vi "SDCP Receiver and Transmitter - Tx Table.vi"(5 "Cell Position":T2, 7 "Table Control":refnum<vi>, 8 "error in (no error)":errorcluster, 9 "Command":T3(ring), 10 "FID":i32, 11 "SMF Parameters descriptors":T4[](array[typedef])) -> (0 "error out":errorcluster, 3 "Table elements out":T1[](array[typedef]))   [LabVIEW 2020]
uses:
  Typedefs/SDCP - SMF parameter descriptors.ctl
  <vilib>/Utility/miscctls.llb/LVRowAndColumnTypeDef.ctl
  Typedefs/SDCP SMF Receiver and Transmitter - Transmit Table Element.ctl
  Typedefs/SDCP - Standard Message Frame Parameters - FGV - commands.ctl
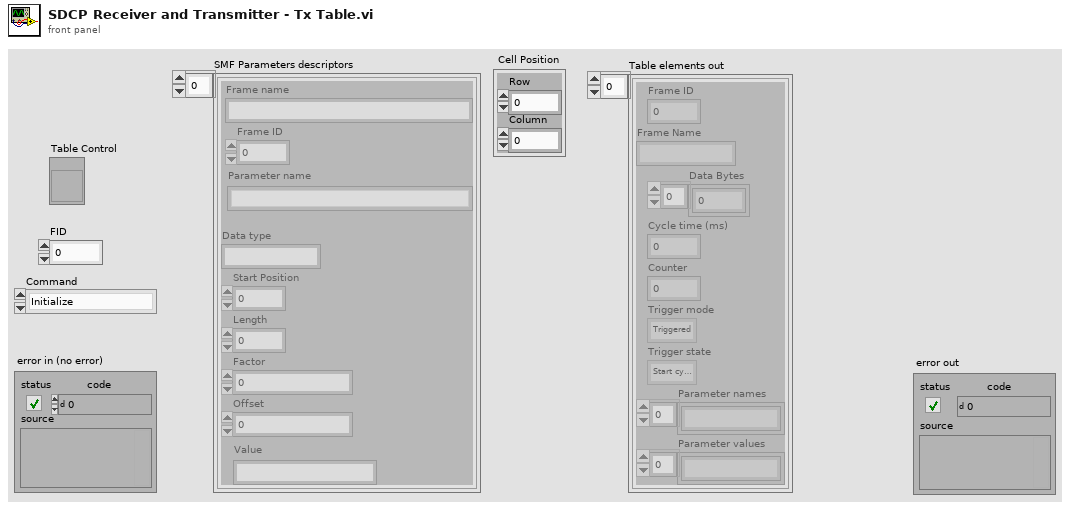
[diagram p1: front panel]
types:
  T1 = typedef "SDCP SMF Receiver and Transmitter - Transmit Table Element.ctl" = cluster{"Frame ID":i32, "Frame Name":string, "Data Bytes":u8[], "Cycle time (ms)":i32, "Counter":i32, "Trigger mode":enum16{"Triggered", "Cyclic"}, "Trigger state":enum16{"Stop cyclic trigger", "Start cyclic trigger", "Stop single trigger", "Start single trigger"}, "Parameter names":string[], "Parameter values":string[]}
  T2 = typedef "LVRowAndColumnTypeDef.ctl" = cluster{"Row":i32, "Column":i32}
  T3 = enum16{"Initialize", "Add row", "Remove row", "Update"}
  T4 = typedef "SDCP - SMF parameter descriptors.ctl" = cluster{"Frame name":string, "Frame ID":i32, "Data type":string, "Start Position":i32, "Length":i32, "Factor":dbl, "Offset":dbl, "Parameter name":string, "Value":string}
  T5 = enum16{"Stop cyclic trigger", "Start cyclic trigger", "Stop single trigger", "Start single trigger"}
  T6 = typedef "SDCP - Standard Message Frame Parameters - FGV - commands.ctl" = enum16{"Write descriptors", "Read descriptors", "Read values", "Load parameters from file", "Write values", "Read all descriptors"}
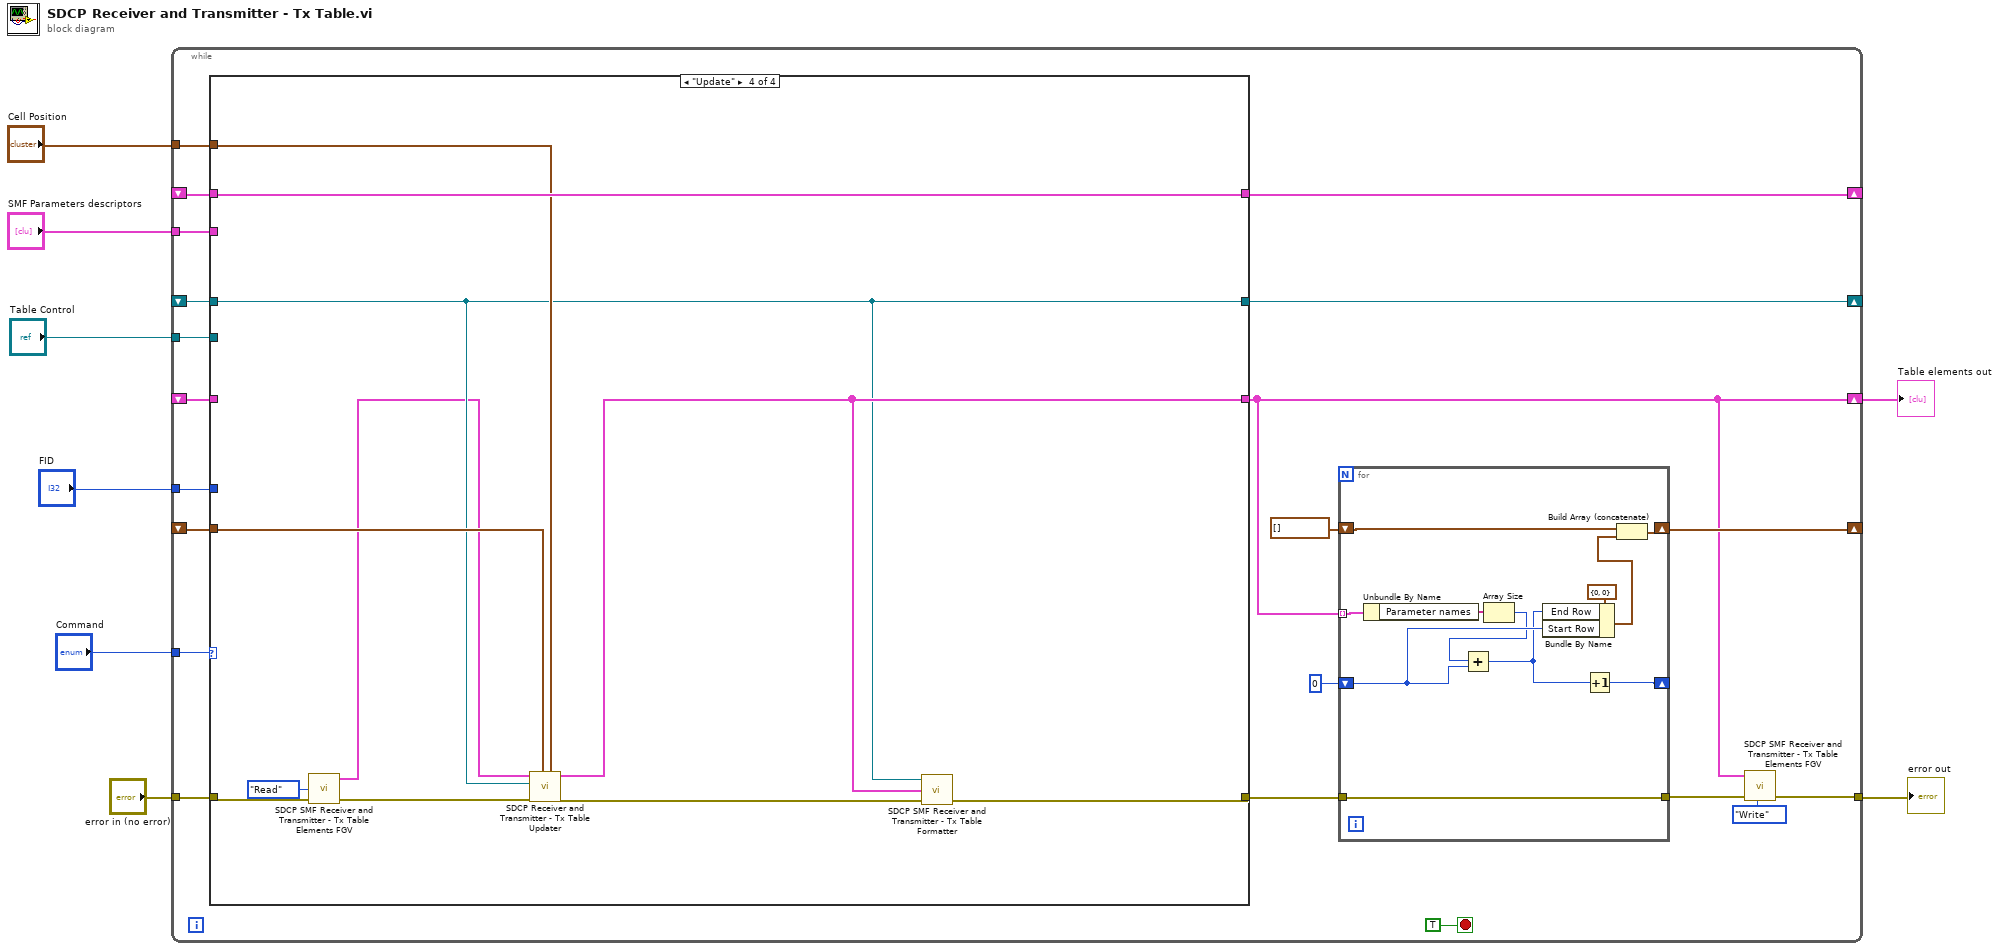
[diagram p0: block diagram]
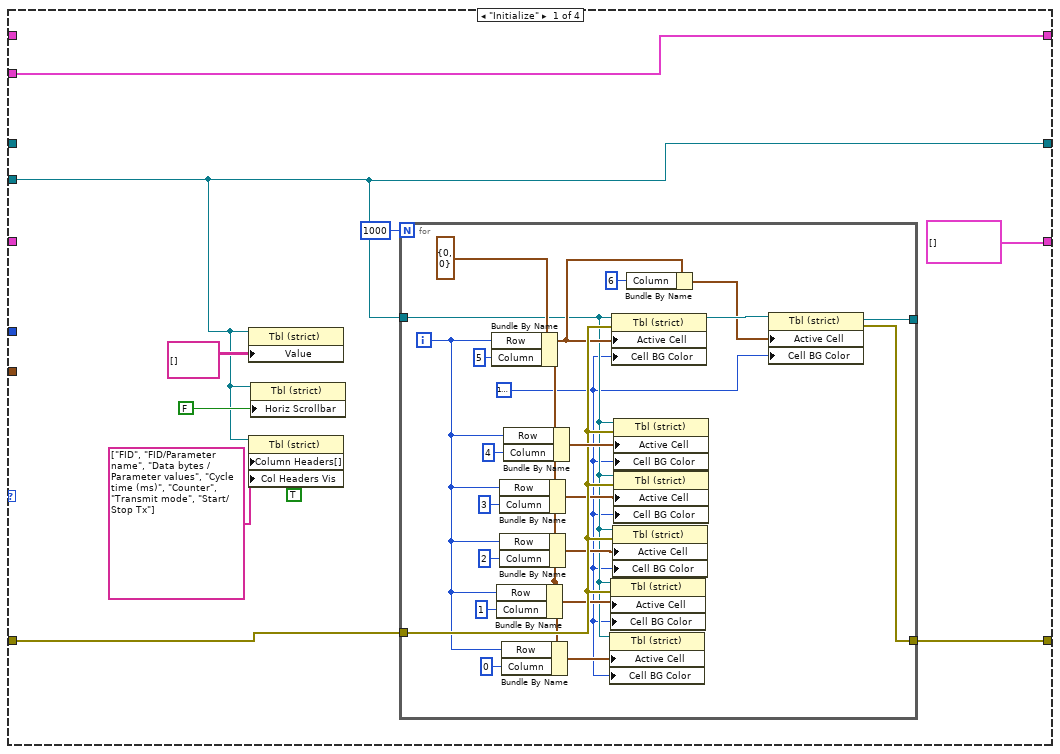
[diagram p2: hidden frame]
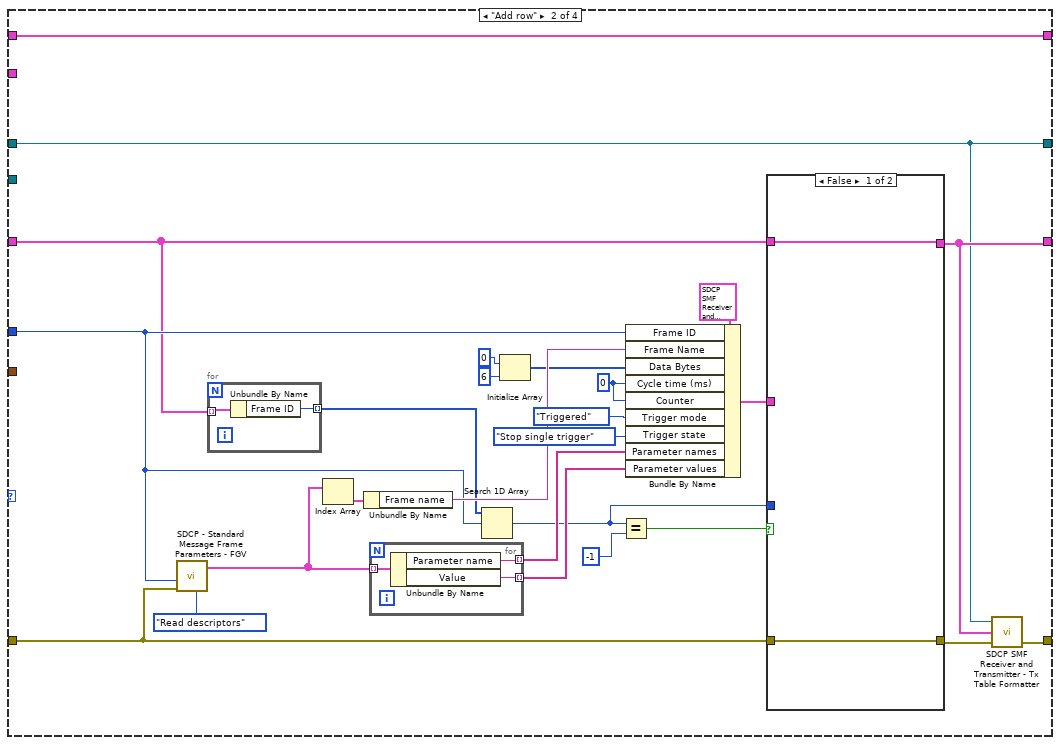
[diagram p3: hidden frame]
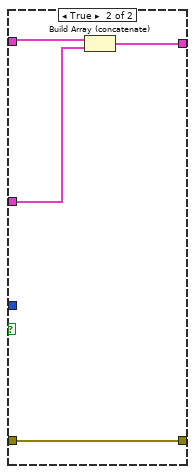
[diagram p4: hidden frame]
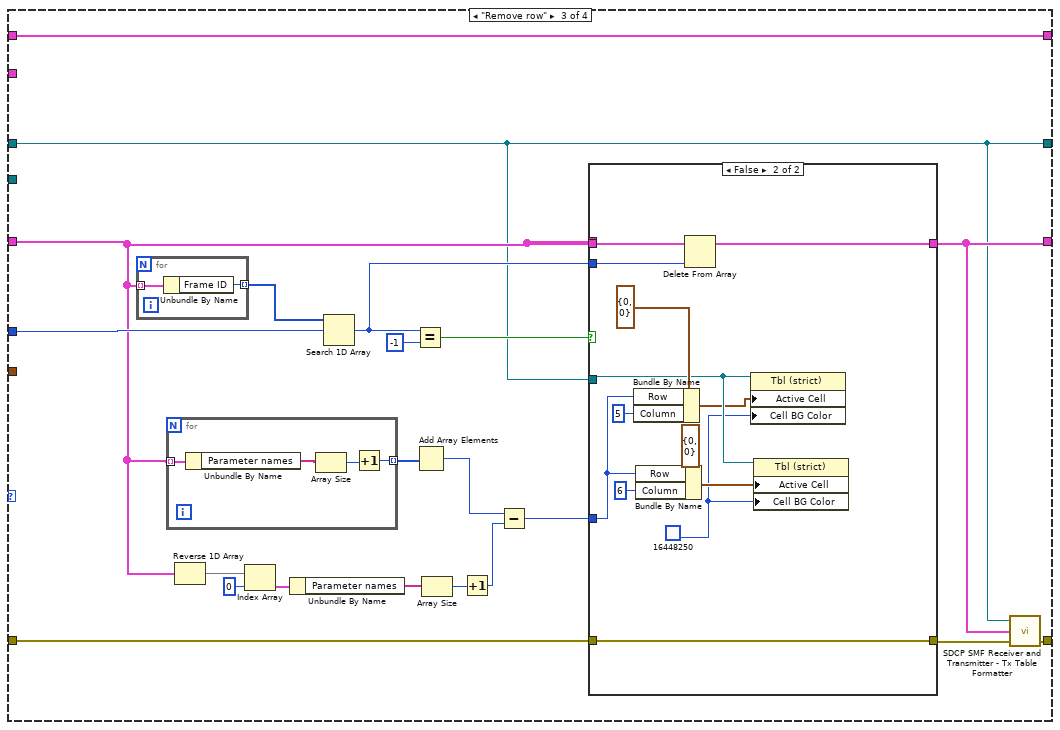
[diagram p5: hidden frame]
diagram:
  n1 = while {
    tunnel: "error in (no error)" -> [w28]
    tunnel: "SMF Parameters descriptors" -> [w27]
    shift-right: [w25] -> _
    shift-left: _ -> [w26]
    tunnel: [w11] -> w6
    shift-right: [w23] -> _
    shift-left: _ -> [w24]
    tunnel: "Table Control" -> [w22]
    tunnel: "Command" -> [w21]
    shift-right: [w10] -> w1
    shift-left: _ -> [w20]
    tunnel: "FID" -> [w19]
    shift-right: [w16] -> _
    shift-left: _ -> [w14]
    tunnel: "Cell Position" -> [w15]
    stop <- TRUE stop-if-true
    n2 = case shown="\"Update\"" w21 {
      tunnel: w28 -> [w47 w81 w125 w155]
      tunnel: w27 -> [w50 _ _ _]
      tunnel: w26 -> [_ w98 w130 w162]
      tunnel: [w50 w98 w130 w162] -> w25
      tunnel: [w46 w76 w122 w156] -> w13
      tunnel: w24 -> [_ w74 w110 w157]
      tunnel: [w43 w74 w110 w157] -> w23
      tunnel: w22 -> [w43 _ _ _]
      tunnel: w20 -> [_ w79 w119 _]
      tunnel: w19 -> [_ w87 w128 _]
      tunnel: [T1[] [] w75 w121 w158] -> w10
      tunnel: w15 -> [_ _ _ w160]
      tunnel: w14 -> [_ _ _ w161]
      frame "Initialize" {
        n3 = property class="Tbl (strict)"(reference=w43, "Value"=string[][] [] ("Item Names")) -> ()  [unwired: 1 in, 2 out]
        n4 = property class="Tbl (strict)"(reference=w43, "Column Headers[]"=string[] ["FID", "FID/Parameter name", "Data bytes / Parameter values", "Cycle time (ms)", "Counter", "Transmit mode", "Start/Stop Tx"] ("Column Header Strings[]"), "Col Headers Vis"=TRUE ("Visible Items:Column Headers Visible")) -> ()  [unwired: 1 in, 2 out]
        n5 = property class="Tbl (strict)"(reference=w43, "Horiz Scrollbar"=FALSE ("Visible Items:Horizontal Scrollbar Visible")) -> ()  [unwired: 1 in, 2 out]
        n6 = for {
          N: 1000 -> [_]
          tunnel: w43 -> [w52]
          tunnel: w47 -> [w63]
          tunnel: [w67] -> w46
          tunnel: [w66] -> _
          i -> [w53]
          w51 = u32 16777225
          n7 = Bundle By Name(cluster=T2 {"Row"=0, "Column"=0} ("Active Cell:Active Cell"), "Row"=w53, "Column"=5) -> (w54:T2)
          n8 = Bundle By Name(cluster=w54, "Row"=w53, "Column"=1) -> (w57:T2)
          n9 = Bundle By Name(cluster=w54, "Row"=w53, "Column"=3) -> (w62:T2)
          n10 = Bundle By Name(cluster=w54, "Row"=w53, "Column"=2) -> (w59:T2)
          n11 = Bundle By Name(cluster=w54, "Row"=w53, "Column"=0) -> (w55:T2)
          n12 = Bundle By Name(cluster=w54, "Row"=w53, "Column"=4) -> (w65:T2)
          n13 = property class="Tbl (strict)"(reference=w52, "Active Cell"=w55, "Cell BG Color"=w51) -> ()  [unwired: 1 in, 2 out]
          n14 = property class="Tbl (strict)"(reference=w52, error in=w63, "Active Cell"=w57, "Cell BG Color"=w51) -> ()  [unwired: 2 out]
          n15 = property class="Tbl (strict)"(reference=w52, error in=w63, "Active Cell"=w54, "Cell BG Color"=w51) -> (reference out=w71:refnum<vi>)  [unwired: 1 out]
          n16 = property class="Tbl (strict)"(reference=w52, error in=w63, "Active Cell"=w59, "Cell BG Color"=w51) -> ()  [unwired: 2 out]
          n17 = property class="Tbl (strict)"(reference=w52, error in=w63, "Active Cell"=w65, "Cell BG Color"=w51) -> ()  [unwired: 2 out]
          n18 = property class="Tbl (strict)"(reference=w52, error in=w63, "Active Cell"=w62, "Cell BG Color"=w51) -> ()  [unwired: 2 out]
          n19 = Bundle By Name(cluster=w54, "Column"=6) -> (w68:T2)
          n20 = property class="Tbl (strict)"(reference=w71, "Active Cell"=w68, "Cell BG Color"=w51) -> (reference out=w66:refnum<vi>, error out=w67:errorcluster)  [unwired: 1 in]
        }
      }
      frame "Add row" {
        w89 = 0 ("Cycle time (ms)")
        n21 = call "SDCP - Standard Message Frame Parameters - FGV.vi"("FID"=w87, "error in (no error)"=w81, "Command"=SDCP_-_Standard_Message_Frame_Parameters_-_FGV_-_commands."Read descriptors") -> ("SMF Parameters descriptors out"=w95:T4[])  [unwired: 4 in, 1 out]
        n22 = for {
          tunnel: w79 -> [w100] mode=indexing
          tunnel: [w99] -> w78 mode=indexing
          n23 = Unbundle By Name(w100) -> ("Frame ID"=w99:i32)
        }
        n24 = Index Array(array=w95) -> (element=w94:T4)  [unwired: 1 in]
        n25 = Unbundle By Name(w94) -> ("Frame name"=w93:string)
        n26 = for {
          tunnel: w95 -> [w109] mode=indexing
          tunnel: [w108] -> w86 mode=indexing
          tunnel: [w107] -> w85 mode=indexing
          n27 = Unbundle By Name(w109) -> ("Parameter name"=w108:string, "Value"=w107:string)
        }
        n28 = Search 1D Array(1D array=w78, element=w87) -> (index of element=w80:i32)  [unwired: 1 in]
        n29 = Initialize Array(u8 0, 6 ("dimension size")) -> (w90:u8[])
        n30 = Equal?(x=w80, y=-1) -> (x = y?=w83:bool)
        n31 = Bundle By Name(cluster=T1 {"Frame ID"=0, "Frame Name"="", "Data Bytes"=[], "Cycle time (ms)"=0, "Counter"=0, "Trigger mode"=enum."Cyclic", "Trigger state"=enum."Start cyclic trigger", "Parameter names"=[], "Parameter values"=[]} ("Transmit table element"), "Frame ID"=w87, "Frame Name"=w93, "Data Bytes"=w90, "Cycle time (ms)"=w89, "Counter"=w89, "Trigger mode"=enum16{"Triggered", "Cyclic"}."Triggered", "Trigger state"=T5."Stop single trigger", "Parameter names"=w86, "Parameter values"=w85) -> (w82:T1)
        n32 = case shown="False" w83 {
          tunnel: w79 -> [w101 w106]
          tunnel: [w101 w105] -> w75
          tunnel: w82 -> [_ w104]
          tunnel: w81 -> [w102 w103]
          tunnel: [w102 w103] -> w77
          tunnel: w80 -> [_ _]
          frame False {
          }
          frame True {
            n33 = Build Array (concatenate)(w106, w104) -> (w105:T1[])
          }
        }
        n34 = call "SDCP SMF Receiver and Transmitter - Tx Table Formatter.vi"("error in (no error)"=w77, "Transmit table elements"=w75, "Table Control"=w74) -> ("error out"=w76:errorcluster)  [unwired: 2 in]
      }
      frame "Remove row" {
        n35 = for {
          tunnel: w119 -> [w151] mode=indexing
          tunnel: [w150] -> w129 mode=indexing
          n36 = Unbundle By Name(w151) -> ("Frame ID"=w150:i32)
        }
        n37 = for {
          tunnel: w119 -> [w134] mode=indexing
          tunnel: [w131] -> w120 mode=indexing
          n38 = Unbundle By Name(w134) -> ("Parameter names"=w133:string[])
          n39 = Array Size(array=w133) -> (size(s)=w132:i32)
          n40 = Increment(x=w132) -> (x+1=w131:i32)
        }
        n41 = Reverse 1D Array(array=w119) -> (reversed array=w118:T1[])
        n42 = Index Array(array=w118, index=0) -> (element=w116:T1)
        n43 = Unbundle By Name(w116) -> ("Parameter names"=w115:string[])
        n44 = Search 1D Array(1D array=w129, element=w128) -> (index of element=w124:i32)  [unwired: 1 in]
        n45 = Equal?(x=w124, y=-1) -> (x = y?=w126:bool)
        n46 = Add Array Elements(numeric array=w120) -> (sum=w114:i32)
        n47 = Array Size(array=w115) -> (size(s)=w113:i32)
        n48 = Increment(x=w113) -> (x+1=w112:i32)
        n49 = Subtract(x=w114, y=w112) -> (x-y=w111:i32)
        n50 = case shown="False" w126 {
          tunnel: w125 -> [w135 w149]
          tunnel: [w135 w149] -> w123
          tunnel: w119 -> [w136 _]
          tunnel: w119 -> [_ w148]
          tunnel: w124 -> [_ w147]
          tunnel: [w136 w146] -> w121
          tunnel: w111 -> [_ w142]
          tunnel: w110 -> [_ w140]
          frame True {
          }
          frame False {
            w137 = u32 16448250
            n51 = Bundle By Name(cluster=T2 {"Row"=0, "Column"=0} ("Active Cell:Active Cell"), "Row"=w142, "Column"=5) -> (w139:T2)
            n52 = Bundle By Name(cluster=T2 {"Row"=0, "Column"=0} ("input cluster"), "Row"=w142, "Column"=6) -> (w138:T2)
            n53 = Delete From Array(array=w148, index=w147) -> (array with subset deleted=w146:T1[])  [unwired: 1 in, 1 out]
            n54 = property class="Tbl (strict)"(reference=w140, "Active Cell"=w139, "Cell BG Color"=w137) -> ()  [unwired: 1 in, 2 out]
            n55 = property class="Tbl (strict)"(reference=w140, "Active Cell"=w138, "Cell BG Color"=w137) -> ()  [unwired: 1 in, 2 out]
          }
        }
        n56 = call "SDCP SMF Receiver and Transmitter - Tx Table Formatter.vi"("error in (no error)"=w123, "Transmit table elements"=w121, "Table Control"=w110) -> ("error out"=w122:errorcluster)  [unwired: 2 in]
      }
      frame "Update" {
        n57 = call "SDCP SMF Receiver and Transmitter - Tx Table Elements FGV.vi"("error in (no error)"=w155, "Command"=enum16{"Read", "Write"}."Read") -> ("error out"=w154:errorcluster, "Table elements out"=w152:T1[])  [unwired: 2 in]
        n58 = call "SDCP Receiver and Transmitter - Tx Table Updater.vi"("Current Cell Position"=w160, "Entry position descriptors"=w161, "error in (no error)"=w154, "Table Control"=w157, "Tx Table entry cluster array in"=w152) -> ("error out"=w159:errorcluster, "Tx Table entry cluster array out"=w158:T1[])  [unwired: 5 in]
        n59 = call "SDCP SMF Receiver and Transmitter - Tx Table Formatter.vi"("error in (no error)"=w159, "Transmit table elements"=w158, "Table Control"=w157) -> ("error out"=w156:errorcluster)  [unwired: 2 in]
      }
    }
    n60 = for {
      shift-right: [w35] -> w16
      shift-left: cluster{"Start Row":i32, "End Row":i32}[] [] -> [w36]
      tunnel: w10 -> [w40] mode=indexing
      shift-right: [w37] -> _
      shift-left: 0 -> [w33]
      tunnel: w13 -> [w30]
      tunnel: [w30] -> w12
      n61 = Unbundle By Name(w40) -> ("Parameter names"=w39:string[])
      n62 = Array Size(array=w39) -> (size(s)=w32:i32)
      n63 = Add(x=w32, y=w33) -> (x+y=w31:i32)
      n64 = Bundle By Name(cluster=cluster{"Start Row":i32, "End Row":i32} {"Start Row"=0, "End Row"=0}, "End Row"=w31, "Start Row"=w33) -> (w34:cluster{"Start Row":i32, "End Row":i32})
      n65 = Increment(x=w31) -> (x+1=w37:i32)
      n66 = Build Array (concatenate)(w36, w34) -> (w35:cluster{"Start Row":i32, "End Row":i32}[])
    }
    n67 = call "SDCP SMF Receiver and Transmitter - Tx Table Elements FGV.vi"("error in (no error)"=w12, "Command"=enum16{"Read", "Write"}."Write", "Table elements in"=w10) -> ("error out"=w11:errorcluster)  [unwired: 1 in, 1 out]
  }
  "error out" <- w6
  "Table elements out" <- w1
